vi "Read Parameters to process.vi"(8 "error in":errorcluster, 11 "ExampleSequencer runtime in":refnum<class "ExampleSequencer runtime.lvclass">) -> (0 "error out":errorcluster, 2 "Parameters to process":T1, 3 "ExampleSequencer runtime out":refnum<class "ExampleSequencer runtime.lvclass">)   [LabVIEW 2017, in "ExampleSequencer runtime.lvclass"]
uses:
  ExampleSequencer runtime.lvclass
  configuration/parameter data indices.ctl
  ExampleSequencer runtime.lvclass/ExampleSequencer runtime.ctl
  configuration/ExampleSequencer configuration.lvclass
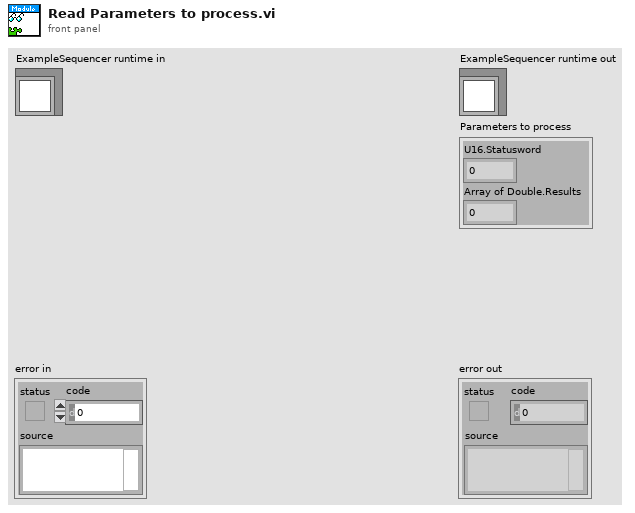
[diagram p1: front panel]
types:
  T1 = typedef "ExampleSequencer configuration.lvclass/parameter data indices.ctl" = cluster{"U16.Statusword":i32, "Array of Double.Results":i32}
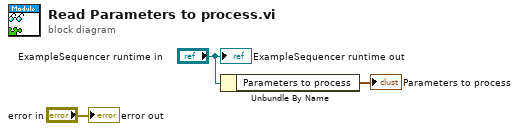
[diagram p0: block diagram]
diagram:
  n1 = Unbundle By Name("ExampleSequencer runtime in") -> ("Parameters to process"=→"Parameters to process":T1)
  "error out" <- "error in"
  "ExampleSequencer runtime out" <- "ExampleSequencer runtime in"
